vi "Waveform - XY Pairs.vi"() -> ()   [LabVIEW 2023]
doc: "Shows how to convert waveform data to XY data with the Waveform to XY Pairs VI."
uses:
  <vilib>/Waveform/WDTOps.llb/WDT Waveform to XY Pairs DBL.vi
panel:
  out "Sine (XY Graph)":cluster{"x":timestamp, "y":dbl}[](graph)
  out "Sine (Waveform Graph)":waveform(dbl)(graph)
  # "Overview: Demonstrates how to convert waveform data to XY data with the Waveform to XY Pairs VI.\nInstructions:\nRun the VI. A sine waveform is displayed in the Sine (Waveform Graph) indicator. That same data is also displayed as XY data in the Sine (XY Graph) indicator."
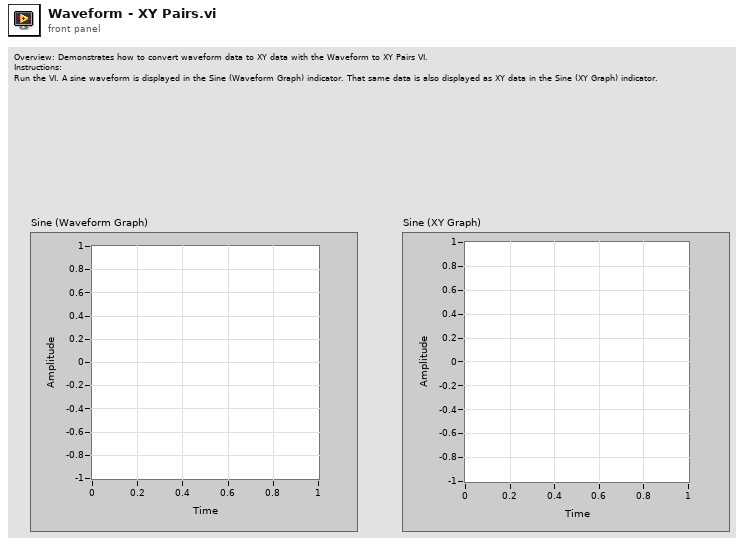
[diagram p1: front panel]
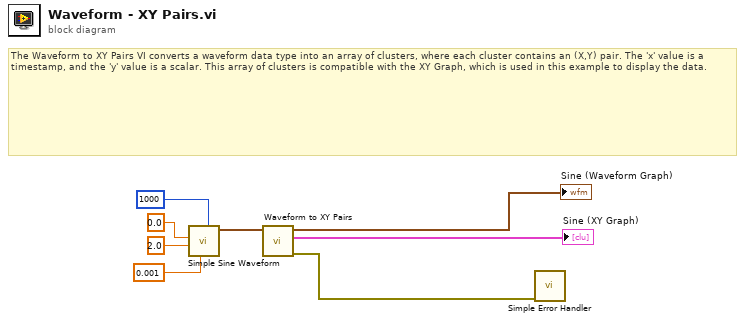
[diagram p0: block diagram]
diagram:
  # "The Waveform to XY Pairs VI converts a waveform data type into an array of clusters, where each cluster contains an (X,Y) pair. The 'x' value is a timestamp, and the 'y' value is a scalar. This array of clusters is compatible with the XY Graph, which is used in this example to display the data."
  n1 = call "Simple Sine Waveform.vi"("n points"=1000, "delta t"=0.001, "n cycles"=2.0 ("frequency"), "t0"=0.0) -> ("sine waveform"=w8:waveform(dbl))  [unwired: 7 in]
  n2 = call-poly <vilib>:"Waveform to XY Pairs.vi"("waveform in"=w8) -> ("error out"=w3:errorcluster, "XY pairs"=→"Sine (XY Graph)":cluster{"x":timestamp, "y":dbl}[], "waveform out"=→"Sine (Waveform Graph)":waveform(dbl))  [unwired: 8 in]
  n3 = call <vilib>:"Simple Error Handler.vi"("error in (no error)"=w3) -> ()  [unwired: 4 in, 5 out]
